vi "FGV_Preis.vi"(7 "fgv-Status":T1, 8 "error in (no error)":errorcluster, 10 "Preis":dbl format="%#_13g") -> (0 "error out":errorcluster, 2 "Preis output":dbl)   [LabVIEW 2023]
doc: "FGV Preis"
uses:
  Pusterhofer/CONTROLS/FGV Status.ctl
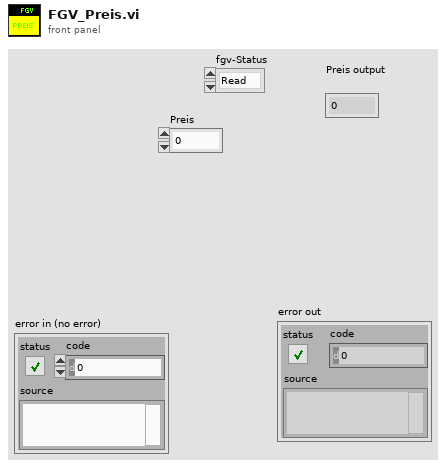
[diagram p1: front panel]
types:
  T1 = typedef "FGV Status.ctl" = enum16{"Read", "Write", ""}
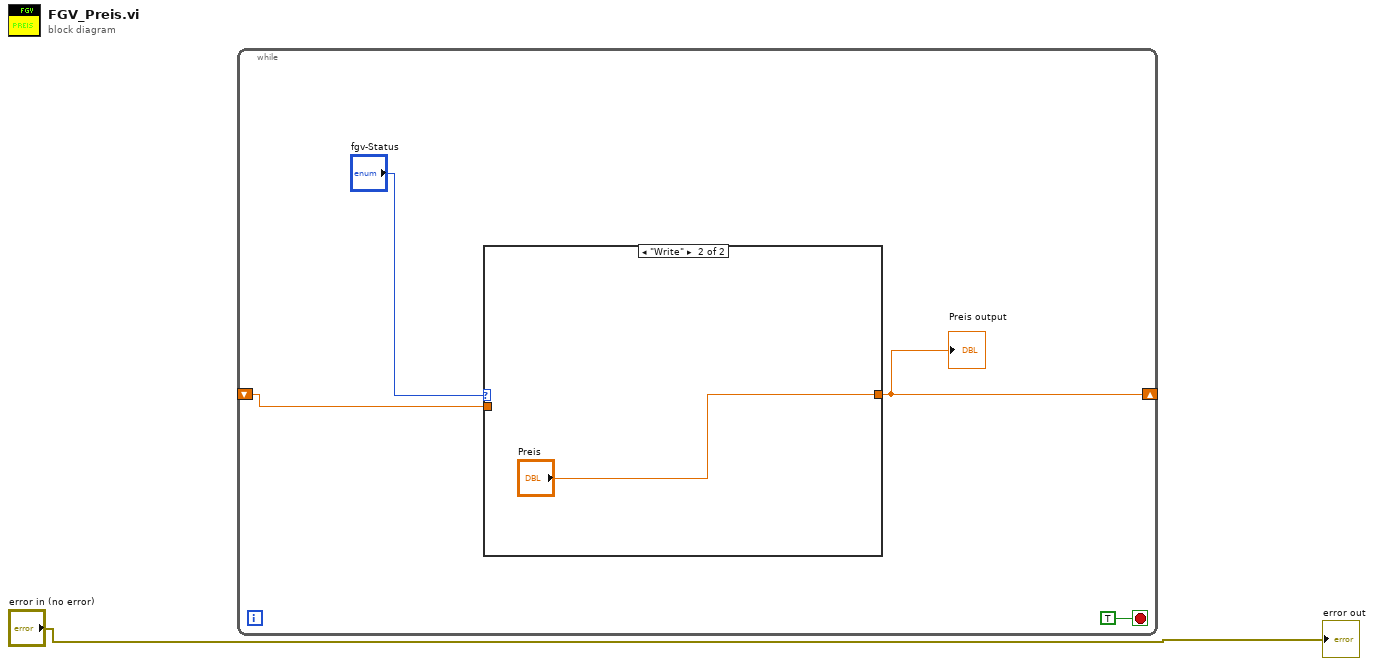
[diagram p0: block diagram]
diagram:
  n1 = while {
    shift-right: [w2] -> _
    shift-left: _ -> [w3]
    stop <- TRUE stop-if-true
    n2 = case shown="\"Write\"" "fgv-Status" {
      tunnel: [w6 "Preis"] -> w2
      tunnel: w3 -> [w6 _]
      frame "Read", Default {
      }
      frame "Write" {
      }
    }
    "Preis output" <- w2
  }
  "error out" <- "error in (no error)"
